vi "LEDDebugColorSwerve.vi"(1 "Shifter State":bool, 2 "Drive Velocity (ft/s)":dbl, 3 "Azimuth Angle (deg [-180,180])":dbl, 4 "Swerve LED Length":i32=4) -> (0 "Color Array":u32[](array[numeric]))   [LabVIEW 2023]
doc: "Sets the LED hue based on the swerve azimuth angle and the intensity based on the swerve drive speed."
uses:
  GlobalDrivebase.vi
  <vilib>/vision/NI_Vision_Development_Module.lvlib
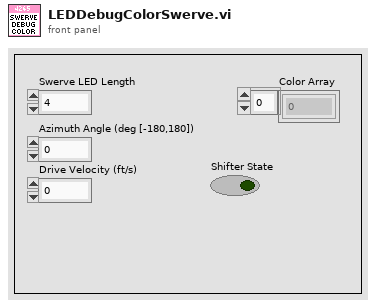
[diagram p1: front panel]
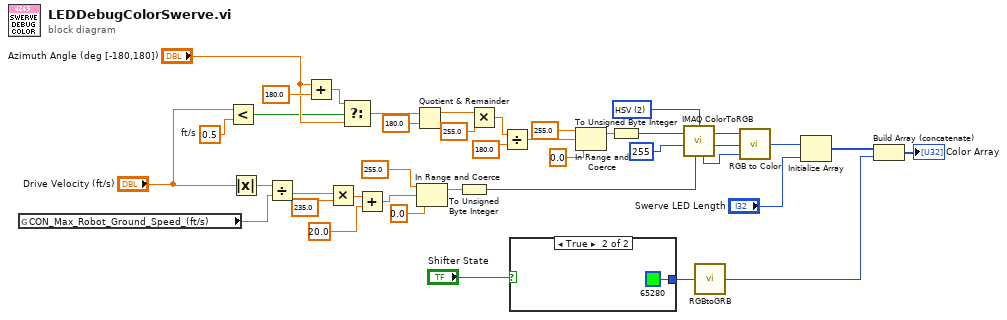
[diagram p0: block diagram]
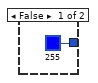
[diagram p2: hidden frame]
diagram:
  w12 = 0.5  # ft/s
  w40 = u16 2 items=["RGB", "HSL", "HSV", "HSI"] ("Color Mode")
  n1 = global read "GlobalDrivebase.vi" "CON_Max_Robot_Ground_Speed_(ft/s)"() -> (w9:dbl)
  n2 = Less?(x="Drive Velocity (ft/s)", y=w12) -> (x < y?=w2:bool)
  n3 = Absolute Value(x="Drive Velocity (ft/s)") -> (abs(x)=w31:dbl)
  n4 = Divide(x=w31, y=w9) -> (x/y=w36:dbl)
  n5 = Add(x="Azimuth Angle (deg [-180,180])", y=180.0) -> (x+y=w27:dbl)
  n6 = Multiply(x=w36, y=235.0) -> (x*y=w14:dbl)
  n7 = Select(t=w27, s=w2, f="Azimuth Angle (deg [-180,180])") -> (s? t:f=w26:dbl)
  n8 = Add(x=w14, y=20.0) -> (x+y=w16:dbl)
  n9 = Quotient & Remainder(x=w26, y=180.0) -> (x-y*floor(x/y)=w24:dbl)  [unwired: 1 out]
  n10 = In Range and Coerce(upper limit=255.0, x=w16, lower limit=0.0) -> (coerced(x)=w32:dbl)  [unwired: 1 out]
  n11 = To Unsigned Byte Integer(number=w32) -> (unsigned 8bit integer=w10:u8)
  n12 = Multiply(x=w24, y=255.0) -> (x*y=w23:dbl)
  n13 = Divide(x=w23, y=180.0) -> (x/y=w20:dbl)
  n14 = case shown="True" "Shifter State" {
    tunnel: [u32 255 ("Color") u32 65280 ("Color")] -> w4
    frame False {
    }
    frame True {
    }
  }
  n15 = In Range and Coerce(upper limit=255.0, x=w20, lower limit=0.0) -> (coerced(x)=w19:dbl)  [unwired: 1 out]
  n16 = To Unsigned Byte Integer(number=w19) -> (unsigned 8bit integer=w18:u8)
  n17 = call "IMAQ ColorToRGB"("Green or Sat value"=u8 255, "Blue or Luma or Val or Inten value"=w10, "Red or Hue value"=w18, "Color Mode"=w40) -> ("Blue value"=w37:u8, "Green value"=w38:u8, "Red value"=w39:u8)  [unwired: 1 in, 1 out]
  n18 = call "RGBtoGRB.vi"("Color (RGB)"=w4) -> ("Color (GRB)"=w5:u32)
  n19 = call <vilib>:"RGB to Color.vi"("B"=w37, "G"=w38, "R"=w39) -> ("Color"=w8:u32)
  n20 = Initialize Array(w8, "Swerve LED Length") -> (w6:u32[])
  n21 = Build Array (concatenate)(w6, w5) -> (→"Color Array":u32[])
